vi "TestMAchineEtat.vi"() -> ()   [LabVIEW 2015]
panel:
  in  "stop":bool
  out "Boolean 2":bool
  in  "start":bool
  in  "stop":bool
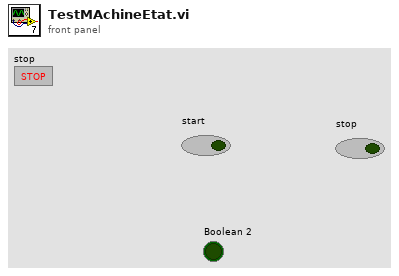
[diagram p1: front panel]
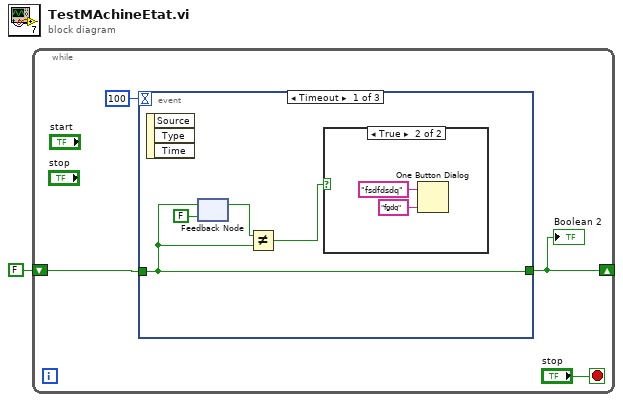
[diagram p0: block diagram]
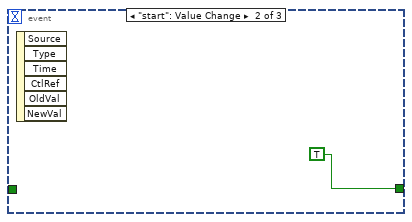
[diagram p3: hidden frame]
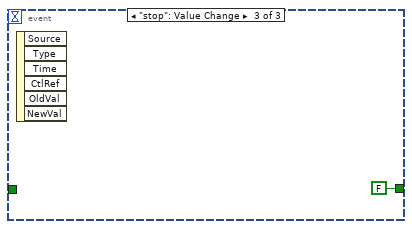
[diagram p4: hidden frame]
diagram:
  n1 = while {
    shift-right: [w2] -> _
    shift-left: FALSE -> [w3]
    stop <- "stop" stop-if-true
    n2 = event shown="[0] Timeout" {
      selector: _ -> [_ _ _]
      dyn-events: _ -> [_ _ _]
      timeout: 100 -> [_ _ _]
      tunnel: [w9 TRUE FALSE] -> w2
      tunnel: w3 -> [w9 _ _]
      event Timeout {
        n3 = event-data() -> ()  [unwired: 1 in, 3 out]
        n4 = feedback-in #1(w9) -> ()
        n5 = feedback #1(FALSE) -> (w7:bool)
        n6 = Not Equal?(x=w7, y=w9) -> (x != y?=w6:bool)
        n7 = case shown="True" w6 {
          frame False {
          }
          frame True {
            n8 = One Button Dialog(message="fsdfdsdq", button name ("OK")="fgdq") -> ()  [unwired: 1 out]
          }
        }
      }
      event "start": Value Change {
        n9 = event-data() -> ()  [unwired: 1 in, 6 out]
      }
      event "stop": Value Change {
        n10 = event-data() -> ()  [unwired: 1 in, 6 out]
      }
    }
    "Boolean 2" <- w2
  }
